vi "HEWH T and Q Max.vi"(0 "UEF Calculated Values":T1 {"Data Indexes"."15 sec after Draw Index" format="%#.2f"; "Data Indexes"."15 sec after Draw Timestamp" format="%#.2f"; "Data Indexes"."Test Start Timestamp" format="%.2f"; "Data Indexes"."Test End Timestamp" format="%.2f"; "Data Indexes"."T0 Timestamp" format="%.2f"; "Data Indexes"."Tsf Timestamp" format="%.2f"; "Data Indexes"."Tsu0 Timestamp" format="%.2f"; "Data Indexes"."Tmax1 Timestamp" format="%.2f"; "Data Indexes"."Draw Index Timestamp" format="%#.2f"; "Data Indexes"."Non-Draw Timestamp" format="%#.2f"; "Data Indexes"."Heating Timestamp" format="%#.2f"; "Data Indexes"."Start Energy (BTU-Gas)" format="%.6f"; "Data Indexes"."Start Watt Hours" format="%.6f"; "Static Data"."V - Volume of Wh (True)" format="%.5f"; "Static Data"."T-Ambinet Nominal (°F)" format="%.5f"; "Static Data"."T-Inlet Setpoint (°F)" format="%.5f"; "Static Data"."T-Wh Setpoint (°F)" format="%.5f"; "Sampled Data"."Qe (Wh)" format="%.5f"; "Sampled Data"."Tau stby2 (hr)" format="%.5f"; "Sampled Data"."Tastby2 (°F)" format="%.5f"; "Sampled Data"."Qf (BTU)" format="%.5f"; "Sampled Data"."Qe (BTU)" format="%.5f"; "Sampled Data"."Tmax1 (°F)" format="%.5f"; "Sampled Data"."T0 (°F)" format="%.5f"; "Sampled Data"."Qr (BTU)" format="%.5f"; "Sampled Data"."T 24(°F)" format="%.5f"; "Sampled Data"."T astby(°F)" format="%.5f"; "Sampled Data"."T tstby(°F)" format="%.5f"; "Sampled Data"."T su0(°F)" format="%.5f"; "Sampled Data"."T suf(°F)" format="%.5f"; "Sampled Data"."Tau stby_1 (hr)" format="%.5f"; "Sampled Data"."Qsuf (BTU)" format="%.5f"; "Sampled Data"."Qsu0 (BTU)" format="%.5f"; "Calculated Values"."Draw Bonus Volume (gal)" format="%.6f"; "Calculated Values"."Adjustment Factor" format="%.6f"; "Calculated Values"."T*avg_del(n-1)" format="%.6f"; "Calculated Values"."T*min(n-1)" format="%.6f"; "Calculated Values"."T*avg_del(n)" format="%.6f"; "Calculated Values"."Vn" format="%.6f"; "Calculated Values"."Qdm (BTU)" format="%.6f"; "Calculated Values"."QHWD (BTU)" format="%.6f"; "Calculated Values"."QHW (BTU)" format="%.6f"; "Calculated Values"."UEF" format="%.6f"; "Calculated Values"."QHW67 (BTU)" format="%.6f"; "Calculated Values"."Qda (BTU)" format="%.6f"; "Calculated Values"."Qd (BTU)" format="%.6f"; "Calculated Values"."Q (BTU)" format="%.6f"; "Calculated Values"."UA (BTU/(hr*F))" format="%.6f"; "Calculated Values"."Qhr (BTU/hr)" format="%.6f"; "Calculated Values"."Qstby (BTU)" format="%.6f"; "Calculated Values"."nu_r" format="%.6f"; "Calculated Values"."CpUEF (BTU/(lb*F))" format="%.6f"; "Calculated Values"."rho_nu (lb/gal)" format="%.6f"; "Calculated Values"."V1- Vol (Gal)" format="%.6f"; "Calculated Values"."M cluster mass removed (lb)" format="%.6f"; "Calculated Values"."Cp theoretical (BTU/(lbm °F))" format="%.6f"; "Calculated Values"."Tin1 - Mean Inlet 1st Cluster (°F)" format="%.6f"; "Calculated Values"."Tdel1-Mean Outlet 1st Cluster(°F)" format="%.6f"; "Calculated Values"."Cp 24 (BTU/(lb*F))" format="%.6f"; "Calculated Values"."Cp standby (BTU/(lb*F))" format="%.6f"; "Calculated Values"."Cp2 (BTU/(lb*F))" format="%.6f"; "Calculated Values"."Cp1 (BTU/(lb*F))" format="%.6f"; "Calculated Values"."rho 24 (lb/gal)" format="%.6f"; "Calculated Values"."rho standby (lb/gal)" format="%.6f"; "Calculated Values"."rho 2 (lb/gal)" format="%.6f"; "Calculated Values"."Density of cold water All (lbm/gal)" format="%#.3g"; "Calculated Values"."CpHW (BTU/(lbm °F))" format="%#.3g"; "Calculated Values"."Density of hot water All (lbm/gal)" format="%#.3g"; "Calculated Values"."Mass of water All (lbm)" format="%#.3f"}, 1 "Watt Hours (String)":dbl[](array[numeric]), 3 "Gas Energy (BTU)":dbl[](array[numeric]), 4 "TC Tree Average":dbl[](array[numeric]), 5 "error in (no error)":errorcluster, 6 "Water Heater Type":T6, 7 "Elapsed Time (sec)":dbl[](array[numeric]), 11 "First Recovery Period Index":i32, 12 "SUf Index":i32) -> (13 "Qsuf":dbl, 14 "UEF Calculated Values Output":T1 {"Data Indexes"."15 sec after Draw Index" format="%#.2f"; "Data Indexes"."15 sec after Draw Timestamp" format="%#.2f"; "Data Indexes"."Test Start Timestamp" format="%.2f"; "Data Indexes"."Test End Timestamp" format="%.2f"; "Data Indexes"."T0 Timestamp" format="%.2f"; "Data Indexes"."Tsf Timestamp" format="%.2f"; "Data Indexes"."Tsu0 Timestamp" format="%.2f"; "Data Indexes"."Tmax1 Timestamp" format="%.2f"; "Data Indexes"."Draw Index Timestamp" format="%#.2f"; "Data Indexes"."Non-Draw Timestamp" format="%#.2f"; "Data Indexes"."Heating Timestamp" format="%#.2f"; "Data Indexes"."Start Energy (BTU-Gas)" format="%.6f"; "Data Indexes"."Start Watt Hours" format="%.6f"; "Static Data"."V - Volume of Wh (True)" format="%.5f"; "Static Data"."T-Ambinet Nominal (°F)" format="%.5f"; "Static Data"."T-Inlet Setpoint (°F)" format="%.5f"; "Static Data"."T-Wh Setpoint (°F)" format="%.5f"; "Sampled Data"."Qe (Wh)" format="%.5f"; "Sampled Data"."Tau stby2 (hr)" format="%.5f"; "Sampled Data"."Tastby2 (°F)" format="%.5f"; "Sampled Data"."Qf (BTU)" format="%.5f"; "Sampled Data"."Qe (BTU)" format="%.5f"; "Sampled Data"."Tmax1 (°F)" format="%.5f"; "Sampled Data"."T0 (°F)" format="%.5f"; "Sampled Data"."Qr (BTU)" format="%.5f"; "Sampled Data"."T 24(°F)" format="%.5f"; "Sampled Data"."T astby(°F)" format="%.5f"; "Sampled Data"."T tstby(°F)" format="%.5f"; "Sampled Data"."T su0(°F)" format="%.5f"; "Sampled Data"."T suf(°F)" format="%.5f"; "Sampled Data"."Tau stby_1 (hr)" format="%.5f"; "Sampled Data"."Qsuf (BTU)" format="%.5f"; "Sampled Data"."Qsu0 (BTU)" format="%.5f"; "Calculated Values"."Draw Bonus Volume (gal)" format="%.6f"; "Calculated Values"."Adjustment Factor" format="%.6f"; "Calculated Values"."T*avg_del(n-1)" format="%.6f"; "Calculated Values"."T*min(n-1)" format="%.6f"; "Calculated Values"."T*avg_del(n)" format="%.6f"; "Calculated Values"."Vn" format="%.6f"; "Calculated Values"."Qdm (BTU)" format="%.6f"; "Calculated Values"."QHWD (BTU)" format="%.6f"; "Calculated Values"."QHW (BTU)" format="%.6f"; "Calculated Values"."UEF" format="%.6f"; "Calculated Values"."QHW67 (BTU)" format="%.6f"; "Calculated Values"."Qda (BTU)" format="%.6f"; "Calculated Values"."Qd (BTU)" format="%.6f"; "Calculated Values"."Q (BTU)" format="%.6f"; "Calculated Values"."UA (BTU/(hr*F))" format="%.6f"; "Calculated Values"."Qhr (BTU/hr)" format="%.6f"; "Calculated Values"."Qstby (BTU)" format="%.6f"; "Calculated Values"."nu_r" format="%.6f"; "Calculated Values"."CpUEF (BTU/(lb*F))" format="%.6f"; "Calculated Values"."rho_nu (lb/gal)" format="%.6f"; "Calculated Values"."V1- Vol (Gal)" format="%.6f"; "Calculated Values"."M cluster mass removed (lb)" format="%.6f"; "Calculated Values"."Cp theoretical (BTU/(lbm °F))" format="%.6f"; "Calculated Values"."Tin1 - Mean Inlet 1st Cluster (°F)" format="%.6f"; "Calculated Values"."Tdel1-Mean Outlet 1st Cluster(°F)" format="%.6f"; "Calculated Values"."Cp 24 (BTU/(lb*F))" format="%.6f"; "Calculated Values"."Cp standby (BTU/(lb*F))" format="%.6f"; "Calculated Values"."Cp2 (BTU/(lb*F))" format="%.6f"; "Calculated Values"."Cp1 (BTU/(lb*F))" format="%.6f"; "Calculated Values"."rho 24 (lb/gal)" format="%.6f"; "Calculated Values"."rho standby (lb/gal)" format="%.6f"; "Calculated Values"."rho 2 (lb/gal)" format="%.6f"; "Calculated Values"."Density of cold water All (lbm/gal)" format="%#.3g"; "Calculated Values"."CpHW (BTU/(lbm °F))" format="%#.3g"; "Calculated Values"."Density of hot water All (lbm/gal)" format="%#.3g"; "Calculated Values"."Mass of water All (lbm)" format="%#.3f"}, 15 "Tsuf":dbl, 16 "End Search Index":i32, 17 "Tsuf Index":i32, 18 "Time @ Index":dbl, 19 "error out":errorcluster)   [LabVIEW 2023]
uses:
  Type Definitions/HEWH Water Heater Type.ctl
  Type Definitions/UEF Constants.ctl
  Type Definitions/HEWH Draw Stats.ctl
  Type Definitions/HEWH FHR Draw Type.ctl
  Type Definitions/FHR Bins.ctl
  Type Definitions/HEWH Meter Type.ctl
panel:
  # "FHR"
  # "FHR"
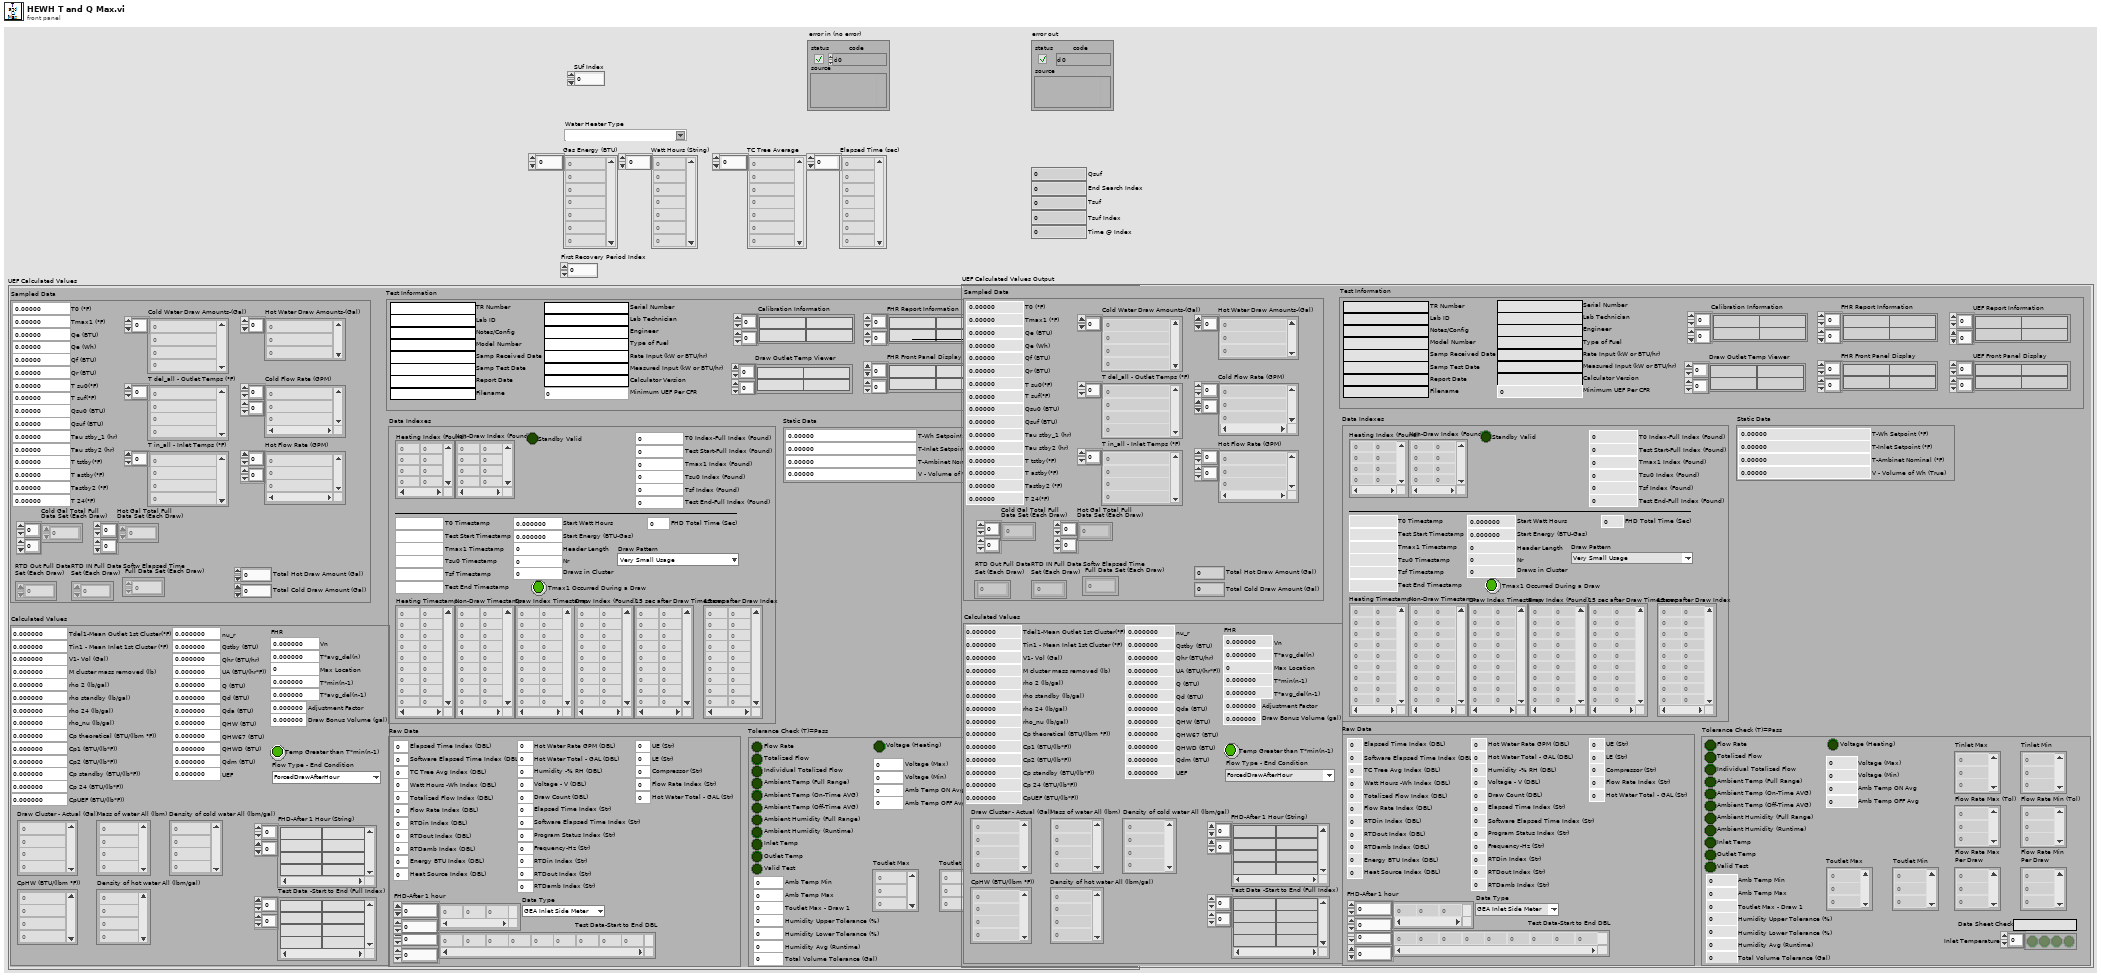
[diagram p1: front panel]
types:
  T1 = typedef "UEF Constants.ctl" = cluster{"Calculated Values":T2, "Sampled Data":cluster{"Cold Water Draw Amounts-(Gal)":dbl[], "T del_all - Outlet Temps (°F)":dbl[], "T in_all - Inlet Temps (°F)":dbl[], "Qsu0 (BTU)":dbl, "Qsuf (BTU)":dbl, "Tau stby_1 (hr)":dbl, "T suf(°F)":dbl, "T su0(°F)":dbl, "T tstby(°F)":dbl, "T astby(°F)":dbl, "T 24(°F)":dbl, "Qr (BTU)":dbl, "T0 (°F)":dbl, "Tmax1 (°F)":dbl, "Qe (BTU)":dbl, "Qf (BTU)":dbl, "Tastby2 (°F)":dbl, "RTD Out Full Data\nSet (Each Draw)":dbl[][], "RTD IN Full Data\nSet (Each Draw)":dbl[][], "Tau stby2 (hr)":dbl, "Hot Water Draw Amounts-(Gal)":dbl[], "Cold Flow Rate (GPM)":dbl[][], "Hot Flow Rate (GPM)":dbl[][], "Softw Elapsed Time\n Full Data Set (Each Draw)":dbl[][], "Cold Gal Total Full\nData Set (Each Draw)":dbl[][], "Total Hot Draw Amount (Gal) ":dbl, "Total Cold Draw Amount (Gal)":dbl, "Qe (Wh)":dbl, "Hot Gal Total Full\nData Set (Each Draw)":dbl[][]}, "Static Data":cluster{"T-Wh Setpoint (°F)":dbl, "T-Inlet Setpoint (°F)":dbl, "T-Ambinet Nominal (°F)":dbl, "V - Volume of Wh (True)":dbl}, "Data Indexes":cluster{"Test Start-Full Index (Found)":i32, "Header Length":i32, "Draw Index (Found)":i32[][], "Nr":i32, "Start Watt Hours":dbl, "Tsu0 Index (Found)":i32, "Tsf Index (Found)":i32, "Start Energy (BTU-Gas)":dbl, "Draws in Cluster":i32, "T0 Index-Full Index (Found)":i32, "Non-Draw Index (Found)":i32[][], "Tmax1 Index (Found)":i32, "Test End-Full Index (Found)":i32, "Heating Index (Found)":i32[][], "Heating Timestamp":dbl[][], "Non-Draw Timestamp":dbl[][], "Draw Index Timestamp":dbl[][], "Tmax1 Timestamp":dbl, "Tsu0 Timestamp":dbl, "Tsf Timestamp":dbl, "T0 Timestamp":dbl, "Test End Timestamp":dbl, "Test Start Timestamp":dbl, "15 sec after Draw Timestamp":dbl[][], "15 sec after Draw Index":dbl[][], "Tmax1 Occurred During a Draw":bool, "FHD Total Time (Sec)":dbl, "Draw Pattern":T4, "Standby Valid":bool}, "Raw Data":cluster{"Elapsed Time Index (DBL)":i32, "Software Elapsed Time Index (DBL)":i32, "TC Tree Avg Index (DBL)":i32, "Watt Hours -Wh Index (DBL)":i32, "Energy BTU Index (DBL)":i32, "Totalized Flow Index (DBL)":i32, "Flow Rate Index (DBL)":i32, "Program Status Index (Str)":i32, "RTDin Index (DBL)":i32, "RTDout Index (DBL)":i32, "RTDamb Index (DBL)":i32, "Test Data-Start to End DBL":dbl[][], "Data Type":T5, "Heat Source Index (DBL)":i32, "Hot Water Rate GPM (DBL)":i32, "Hot Water Total - GAL (DBL)":i32, "FHD-After 1 hour":dbl[][], "Humidity -% RH (DBL)":i32, "Voltage - V (DBL)":i32, "Draw Count (DBL)":i32, "Elapsed Time Index (Str)":i32, "Software Elapsed Time Index (Str)":i32, "Frequency-Hz (Str)":i32, "RTDin Index (Str)":i32, "RTDout Index (Str)":i32, "RTDamb Index (Str)":i32, "UE (Str)":i32, "LE (Str)":i32, "Compressor (Str)":i32, "Flow Rate Index (Str)":i32, "Hot Water Total - GAL (Str)":i32}, "Tolerance Check (T)=Pass":cluster{"Flow Rate":bool, "Totalized Flow":bool, "Ambient Temp (Full Range)":bool, "Ambient Humidity (Full Range)":bool, "Inlet Temp":bool, "Outlet Temp":bool, "Valid Test":bool, "Individual Totalized Flow":bool, "Data Sheet Check":string, "Inlet Temperature":bool[], "Tinlet Max":dbl[], "Tinlet Min":dbl[], "Flow Rate Max (Tol)":dbl[], "Flow Rate Min (Tol)":dbl[], "Amb Temp Max":dbl, "Amb Temp Min":dbl, "Toutlet Max - Draw 1":dbl, "Humidity Upper Tolerance (%)":dbl, "Total Volume Tolerance (Gal)":dbl, "Humidity Lower Tolerance (%)":dbl, "Flow Rate Max\nPer Draw":dbl[], "Flow Rate Min\nPer Draw":dbl[], "Ambient Humidity (Runtime)":bool, "Humidity Avg (Runtime)":dbl, "Ambient Temp (On-Time AVG)":bool, "Ambient Temp (Off-Time AVG)":bool, "Amb Temp OFF Avg":dbl, "Amb Temp ON Avg":dbl, "Voltage (Heating)":bool, "Voltage (Min)":dbl, "Voltage (Max)":dbl, "Toutlet Max":dbl[], "Toutlet Min":dbl[]}, "Test Information":cluster{"TR Number":string, "Lab ID":string, "Notes/Config":string, "Model Number":string, "Serial Number":string, "Lab Technician":string, "Engineer":string, "Type of Fuel":string, "Samp Received Date":string, "Samp Test Date":string, "Report Date":string, "Rate Input (kW or BTU/hr)":string, "Measured Input (kW or BTU/hr)":string, "Filename":string, "Calibration Information":string[][], "Calculator Version":string, "Minimum UEF Per CFR":dbl, "UEF Report Information":string[][], "FHR Report Information":string[][], "FHR Front Panel Display":string[][], "UEF Front Panel Display":string[][], "Draw Outlet Temp Viewer":string[][]}}
  T2 = typedef "HEWH Draw Stats.ctl" = cluster{"Draw Cluster - Actual (Gal)":dbl[], "Mass of water All (lbm)":dbl[], "Density of hot water All (lbm/gal)":dbl[], "CpHW (BTU/(lbm °F))":dbl[], "rho 2 (lb/gal)":dbl, "rho standby (lb/gal)":dbl, "rho 24 (lb/gal)":dbl, "Cp1 (BTU/(lb*F))":dbl, "Cp2 (BTU/(lb*F))":dbl, "Cp standby (BTU/(lb*F))":dbl, "Cp 24 (BTU/(lb*F))":dbl, "nu_r":dbl, "Qstby (BTU)":dbl, "Qhr (BTU/hr)":dbl, "UA (BTU/(hr*F))":dbl, "Q (BTU)":dbl, "Qd (BTU)":dbl, "Qda (BTU)":dbl, "QHW67 (BTU)":dbl, "UEF":dbl, "Tdel1-Mean Outlet 1st Cluster(°F)":dbl, "Tin1 - Mean Inlet 1st Cluster (°F)":dbl, "Cp theoretical (BTU/(lbm °F))":dbl, "M cluster mass removed (lb)":dbl, "V1- Vol (Gal)":dbl, "Test Data -Start to End (Full Index)":string[][], "rho_nu (lb/gal)":dbl, "Density of cold water All (lbm/gal)":dbl[], "CpUEF (BTU/(lb*F))":dbl, "QHW (BTU)":dbl, "QHWD (BTU)":dbl, "Qdm (BTU)":dbl, "FHD-After 1 Hour (String)":string[][], "Vn":dbl, "T*avg_del(n)":dbl, "Max Location":i32, "T*min(n-1)":dbl, "T*avg_del(n-1)":dbl, "Temp Greater than T*min(n-1)":bool, "Adjustment Factor":dbl, "Draw Bonus Volume (gal)":dbl, "Flow Type - End Condition":T3}
  T3 = typedef "HEWH FHR Draw Type.ctl" = enum16{"ForcedDrawAfterHour", "HeatingCutoffBeforeHour"}
  T4 = typedef "FHR Bins.ctl" = enum16{"Very Small Usage", "Low Usage", "Medium Usage", "High Usage", "Undefined"}
  T5 = typedef "HEWH Meter Type.ctl" = enum16{"GEA Inlet Side Meter", "GEA Outlet Side Meter", "CSA Inlet Side Meter"}
  T6 = typedef "HEWH Water Heater Type.ctl" = string
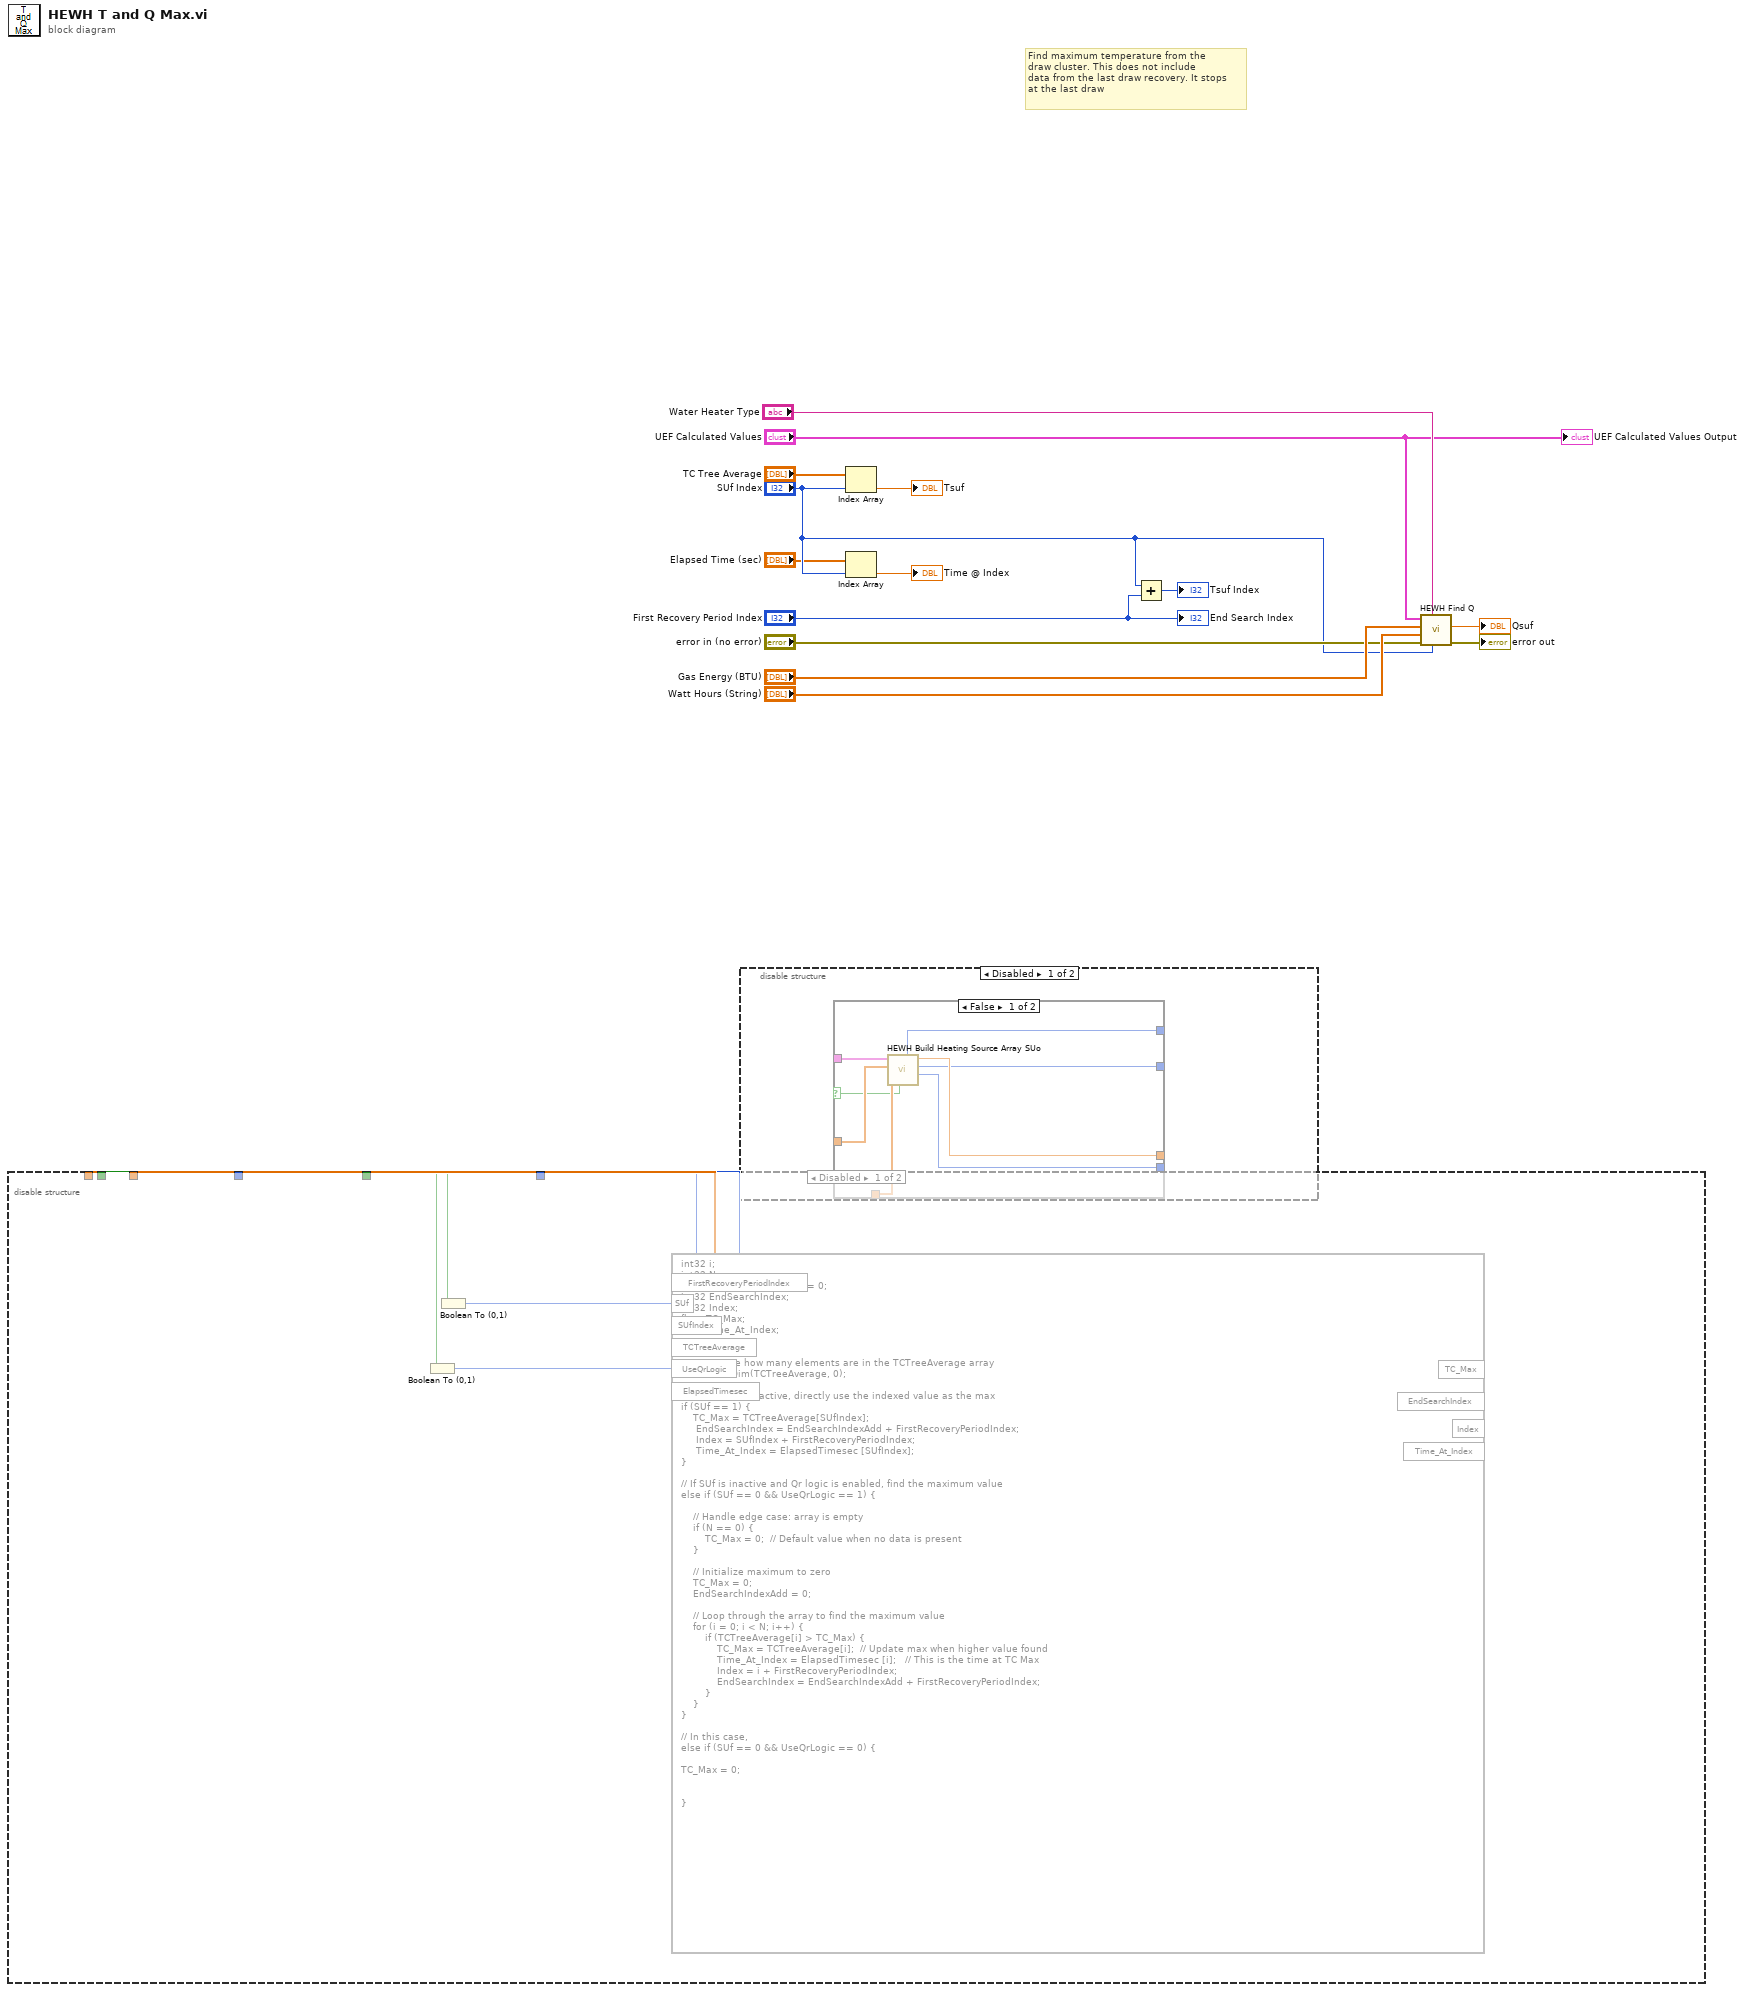
[diagram p0: block diagram]
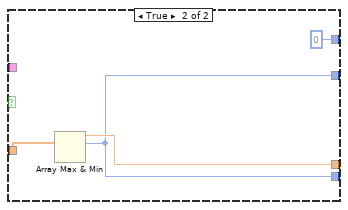
[diagram p2: hidden frame]
diagram:
  # "Find maximum temperature from the \ndraw cluster. This does not include\ndata from the last draw recovery. It stops \nat the last draw"
  n1 = disable-structure shown="Disabled" {
    disable-tunnel: _ -> [w22 _]
    disable-tunnel: _ -> [w21 _]
    disable-tunnel: _ -> [w19 _]
    disable-tunnel: _ -> [w18 _]
    disable-tunnel: _ -> [w16 _]
    disable-tunnel: _ -> [w15 _]
    frame Disabled {
      n2 = Boolean To (0,1)(Boolean=w18) -> (0, 1=w17:i16)
      n3 = Boolean To (0,1)(Boolean=w19) -> (0, 1=w20:i16)
      n4 = formula code="int32 i;\nint32 N;\nint32 EndSearchIndexAdd = 0;\nint32 EndSearchIndex;\nint32 Index;\nfloat TC_Max;\nfloat Time_At_Index;\n\n\n// Determine how many elements are in the TCTreeAverage array\nN = sizeOfDim(TCTreeAverage, 0);\n\n// If SUf mode is active, directly use the indexed value as the max\nif (SUf == 1) {\n    TC_Max = TCTreeAverage[SUfIndex];\n     EndSearchIndex = EndSearchIndexAdd + FirstRecoveryPeriodIndex;\n     Index = SUfIndex + FirstRecoveryPeriodIndex;\n     Time_At_Index = ElapsedTimesec [SUfIndex];\n}\n\n// If SUf is inactive and Qr logic is enabled, find the maximum value\nelse if (SUf == 0 && UseQrLogic == 1) {\n\n    // Handle edge case: array is empty\n    if (N == 0) {\n        TC_Max = 0;  // Default value when no data is present\n    }\n\n    // Initialize maximum to zero\n    TC_Max = 0;\n    EndSearchIndexAdd = 0;\n\n    // Loop through the array to find the maximum value\n    for (i = 0; i < N; i++) {\n        if (TCTreeAverage[i] > TC_Max) {\n            TC_Max = TCTreeAverage[i];  // Update max when higher value found\n            Time_At_Index = ElapsedTimesec [i];   // This is the time at TC Max\n            Index = i + FirstRecoveryPeriodIndex;\n            EndSearchIndex = EndSearchIndexAdd + FirstRecoveryPeriodIndex;\n        }\n    }\n}\n\n// In this case, \nelse if (SUf == 0 && UseQrLogic == 0) {\n\nTC_Max = 0;\n\n\n}"("TCTreeAverage"=w22, "SUfIndex"=w21, "SUf"=w20, "UseQrLogic"=w17, "FirstRecoveryPeriodIndex"=w16, "ElapsedTimesec"=w15) -> ()  [unwired: 4 out]
    }
    frame Enabled {
    }
  }
  n5 = disable-structure shown="Disabled" {
    frame Disabled {
      n6 = case shown="False" {
        selector: _ -> [w23 _]
        tunnel: [w26 w32] -> _
        tunnel: [w27 w34] -> _
        tunnel: _ -> [w29 w33]
        tunnel: _ -> [w30 _]
        tunnel: _ -> [w28 _]
        tunnel: [w25 w32] -> _
        tunnel: [w24 0 ("New End Index")] -> _
        frame False {
          n7 = call "HEWH Build Heating Source Array SUo.vi"("Qr (T), SU0 (F)"=w23, "Elapsed Time (sec)"=w28, "TC Tree Average"=w29, "UEF Calculated Values"=w30) -> ("Subset Index"=w26:i32, "max index(es)"=w25:i32, "max value"=w27:dbl, "New End Index"=w24:i32)  [unwired: 3 in, 1 out]
        }
        frame True {
          n8 = Array Max & Min(array=w33) -> (max value=w34:dbl, max index (indices)=w32:i32)  [unwired: 2 out]
        }
      }
    }
    frame Enabled {
    }
  }
  n9 = Index Array(array="TC Tree Average", index="SUf Index") -> (element=→"Tsuf":dbl)
  n10 = Index Array(array="Elapsed Time (sec)", index="SUf Index") -> (element=→"Time @ Index":dbl)
  n11 = Add(x="SUf Index", y="First Recovery Period Index") -> (x+y=→"Tsuf Index":i32)
  n12 = call "HEWH Find Q.vi"("Q Index"="SUf Index", "Water Heater Type"="Water Heater Type", "error in (no error)"="error in (no error)", "Watt Hours (String)"="Watt Hours (String)", "Gas Energy (BTU)"="Gas Energy (BTU)", "UEF Calculated Values"="UEF Calculated Values") -> ("error out"=→"error out":errorcluster, "Qr (BTU)"=→"Qsuf":dbl)  [unwired: 4 in]
  "UEF Calculated Values Output" <- "UEF Calculated Values"
  "End Search Index" <- "First Recovery Period Index"
